vi "pp2_webcam_test.vi"() -> ()   [LabVIEW 2013]
uses:
  <vilib>/vision/driver/NI_Vision_Acquisition_Software.lvlib
  <vilib>/vision/Image Controls.llb/IMAQ Image.ctl
panel:
  in  "Stop (F) 2":bool caption="Stop (F)"
  out "Image Out 3":T1(plugin-control)
  in  "Stop (F)":bool
  out "Image Out 2":T1(plugin-control)
  in  "Number of Images":i32=20
  out "Image Out":T1(plugin-control)
  out "error out":errorcluster
  out "Image 3":T1(plugin-control)
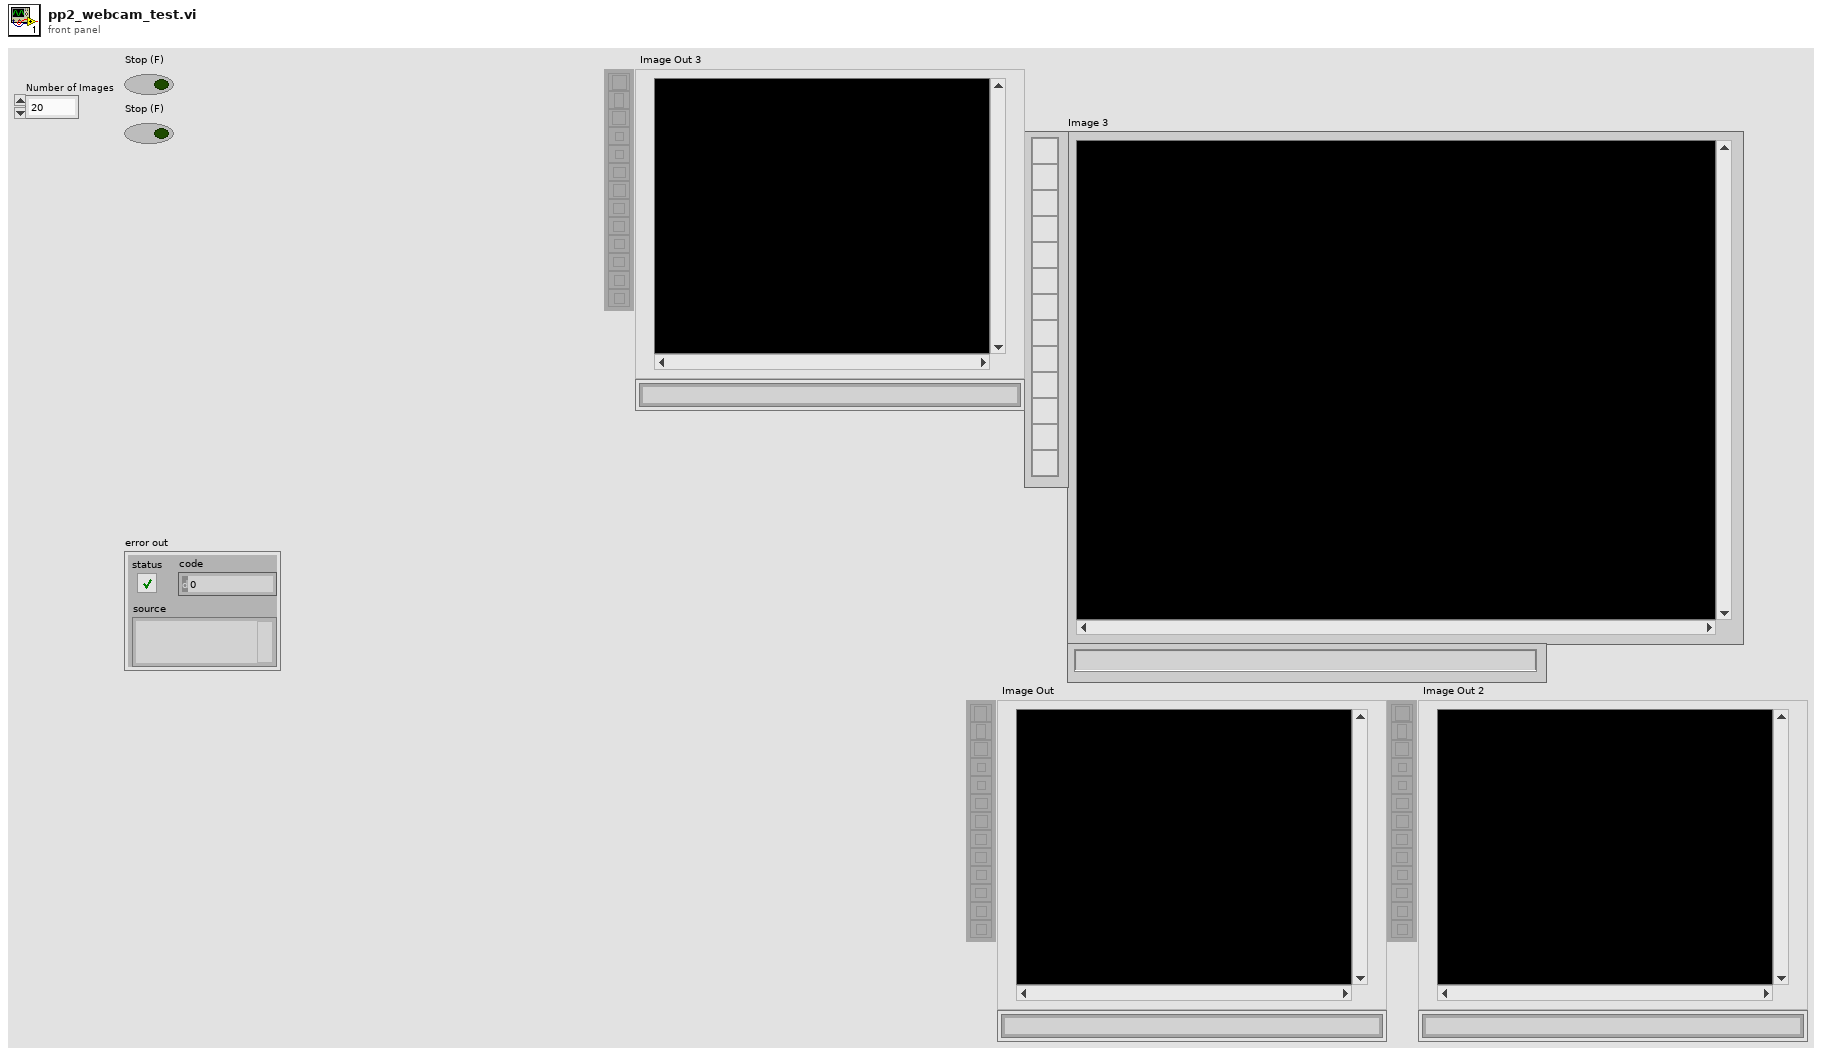
[diagram p1: front panel]
types:
  T1 = typedef "IMAQ Image.ctl" = refnum<image>
  T2 = typedef "IMAQdx.ctl" = refnum<k21>
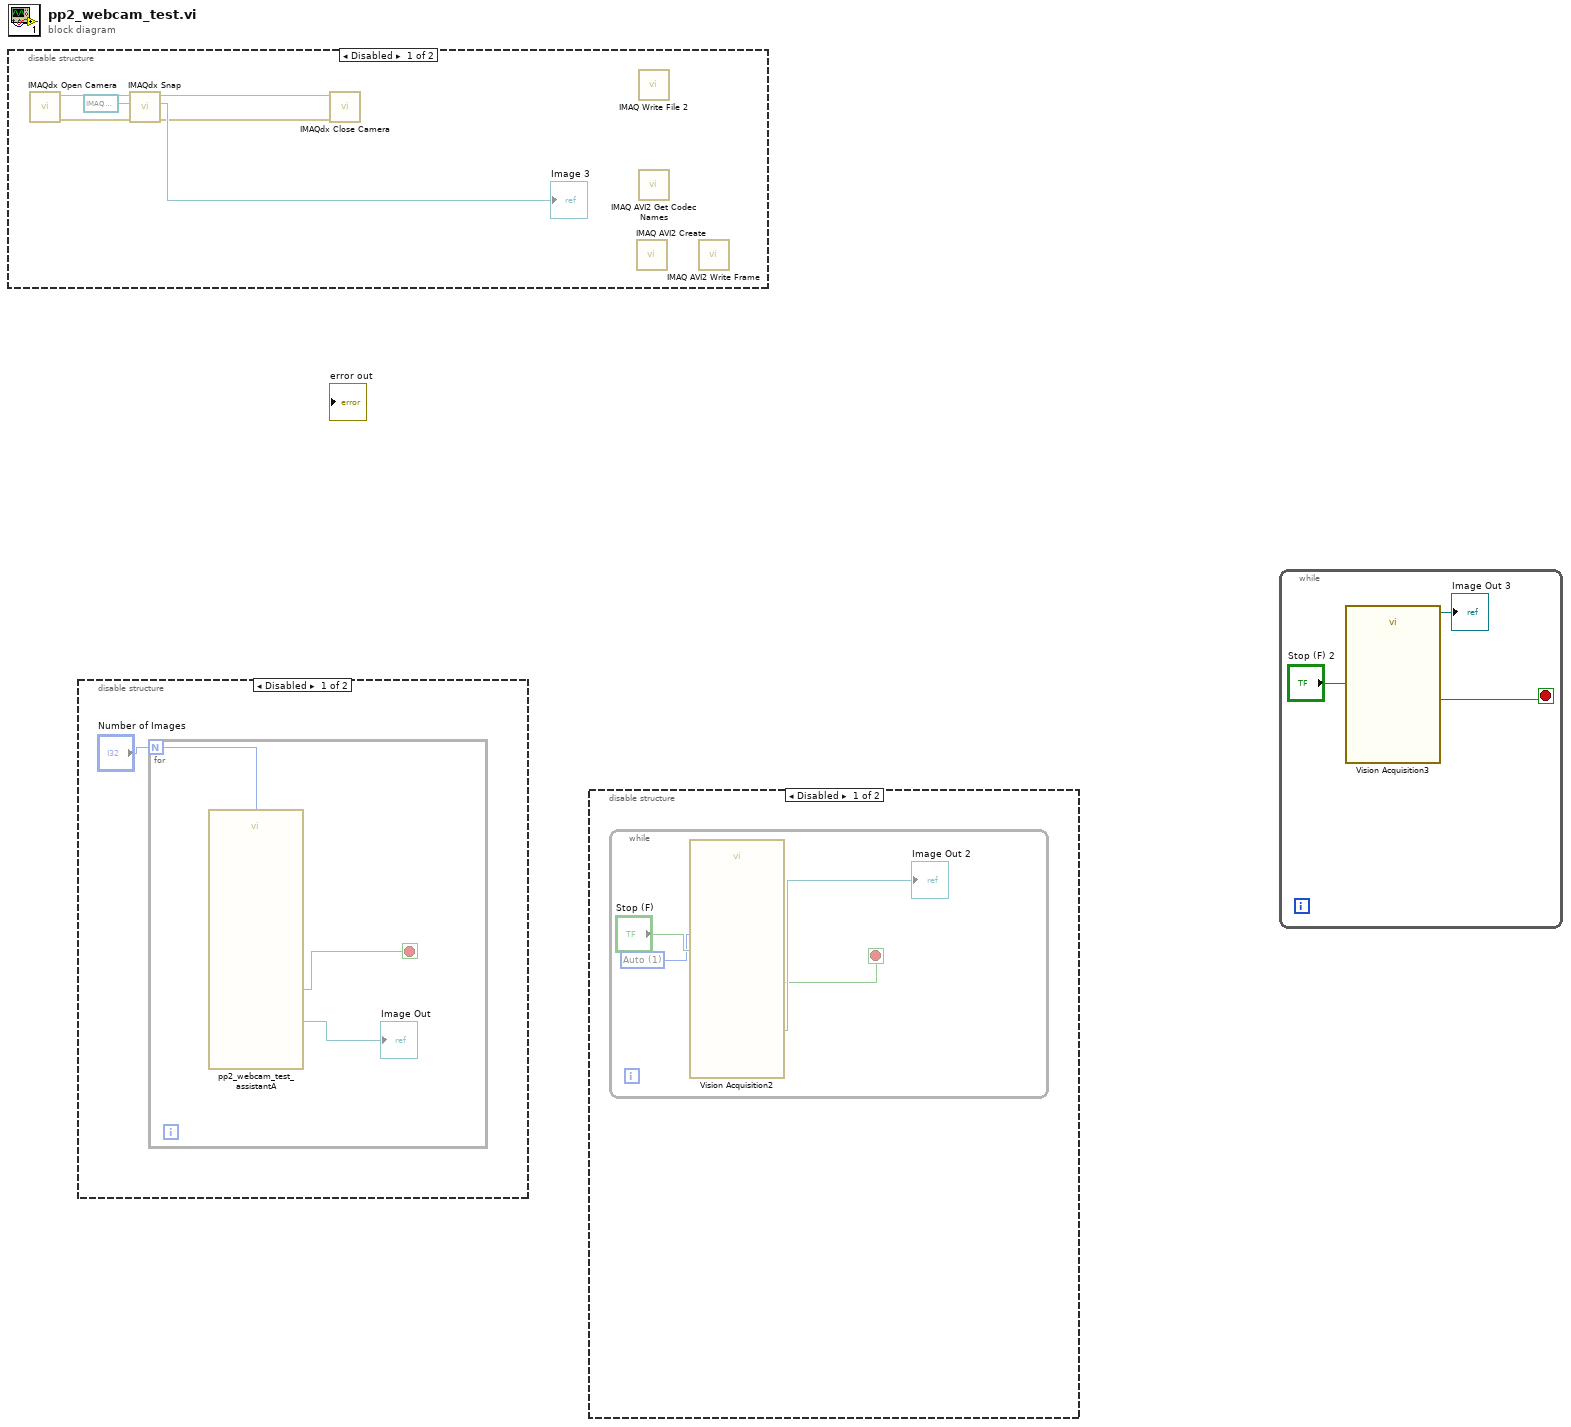
[diagram p0: block diagram]
diagram:
  n1 = disable-structure shown="Disabled" {
    frame Disabled {
      n2 = call <vilib>:"IMAQdx Open Camera.vi"() -> ("error out"=w4:errorcluster, "Session Out"=w5:T2)  [unwired: 10 in]
      n3 = call <vilib>:"IMAQdx Snap.vi"("error in"=w4, "Image In"=T1 refnum, "Session In"=w5) -> ("error out"=w2:errorcluster, "Image Out"=→"Image 3":T1, "Session Out"=w3:T2)  [unwired: 6 in]
      n4 = call <vilib>:"IMAQdx Close Camera.vi"("error in"=w2, "Session In"=w3) -> ()  [unwired: 9 in, 1 out]
      n5 = call "IMAQ AVI2 Create"() -> ()  [unwired: 10 in, 2 out]
      n6 = call-poly "IMAQ Write File 2"() -> ()  [unwired: 10 in, 2 out]
      n7 = call "IMAQ AVI2 Get Codec Names"() -> ()  [unwired: 10 in, 2 out]
      n8 = call "IMAQ AVI2 Write Frame"() -> ()  [unwired: 9 in, 3 out]
    }
    frame Enabled {
    }
  }
  n9 = disable-structure shown="Disabled" {
    frame Disabled {
      n10 = for {
        N: "Number of Images" -> [w9]
        stop <- w8 stop-if-true
        n11 = call "pp2_webcam_test_assistantA.vi"("Number of Images"=w9) -> ("Image Out"=→"Image Out":T1, "Stopped"=w8:bool)  [unwired: 22 in, 3 out]
      }
    }
    frame Enabled {
    }
  }
  n12 = disable-structure shown="Disabled" {
    frame Disabled {
      n13 = while {
        stop <- w12 stop-if-true
        w11 = u32 1 items=["Auto"=1, "Manual"=2] ("Focus::Mode")
        n14 = call "Vision Acquisition2"("Focus::Mode"=w11, "Stop (F)"="Stop (F)") -> ("Image Out"=→"Image Out 2":T1, "Stopped"=w12:bool)  [unwired: 20 in, 4 out]
      }
    }
    frame Enabled {
    }
  }
  n15 = while {
    stop <- w15 stop-if-true
    n16 = call "Vision Acquisition3"("Stop (F)"="Stop (F) 2") -> ("Image Out"=→"Image Out 3":T1, "Stopped"=w15:bool)  [unwired: 24 in, 1 out]
  }
